vi "New ImageData[].vi"(8 "error in (no error)":errorcluster, 10 "ImageData[]":T1[](array[typedef]), 11 "CircularBuffer.ImageData":refnum<class "CircularBuffer.ImageData.lvclass">) -> (0 "error out":errorcluster, 2 "lastElementIndex":i32=1, 3 "CircularBuffer.ImageData out":refnum<class "CircularBuffer.ImageData.lvclass">)   [LabVIEW 2015, in "CircularBuffer.ImageData.lvclass"]
uses:
  CircularBuffer.ImageData.lvclass
  <vilib>/picture/picture.llb/imagedata.ctl
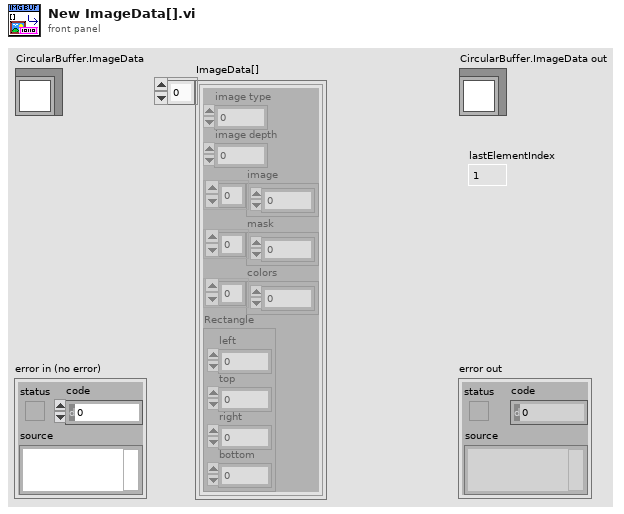
[diagram p1: front panel]
types:
  T1 = typedef "imagedata.ctl" = cluster{"image type":i32, "image depth":i32, "image":u8[], "mask":u8[], "colors":u32[], "Rectangle":cluster{"left":i16, "top":i16, "right":i16, "bottom":i16}}
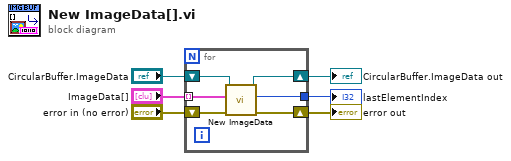
[diagram p0: block diagram]
diagram:
  n1 = for {
    tunnel: [w11] -> w2
    tunnel: "ImageData[]" -> [w12] mode=indexing
    shift-right: [w10] -> w5
    shift-left: "CircularBuffer.ImageData" -> [w9]
    shift-right: [w7] -> w3
    shift-left: "error in (no error)" -> [w8]
    n2 = call "New ImageData.vi"("error in (no error)"=w8, "ImageData"=w12, "CircularBuffer.ImageData"=w9) -> ("error out"=w7:errorcluster, "newElementIndex"=w11:i32, "CircularBuffer.ImageData out"=w10:refnum<class "CircularBuffer.ImageData.lvclass">)  [unwired: 6 in]
  }
  "error out" <- w3
  "CircularBuffer.ImageData out" <- w5
  "lastElementIndex" <- w2
